vi "Config Spark Max SLOT Close Loop HW Get Set.vi"(4 "PIDF Slot (0)":i32, 6 "Get(f) Set(t)":bool, 7 "SparkMax Slot CL":T1={"Gains"={"P"=0.1, "I"=0.0, "D"=0.0, "F"=0.0}, "I Zone"=1.0, "Peak Out -1 0 1"={"High"=0.0, "Low"=0.0}, "Max I Accu"=0.0} {"Gains"."F" format="%#.8f"; "Gains"."D" format="%#.8f"; "Gains"."I" format="%#.8f"; "Gains"."P" format="%#.8f"; "Peak Out -1 0 1"."Low" format="%#.8f"; "Peak Out -1 0 1"."High" format="%#.8f"}, 8 "Error":errorcluster, 11 "Drive Refs":T4) -> (0 "Error Out":errorcluster, 3 "Drive Refs Out":T4, 5 "SparkMax Slot CL Out":T1={"Gains"={"P"=0.1, "I"=0.0, "D"=0.0, "F"=0.0}, "I Zone"=1.0, "Peak Out -1 0 1"={"High"=0.0, "Low"=0.0}, "Max I Accu"=0.0} {"Gains"."F" format="%#.8f"; "Gains"."D" format="%#.8f"; "Gains"."I" format="%#.8f"; "Gains"."P" format="%#.8f"; "Peak Out -1 0 1"."Low" format="%#.8f"; "Peak Out -1 0 1"."High" format="%#.8f"})   [LabVIEW 2020, in "Swerve AM_ACT.lvlib"]
uses:
  Swerve AM_ACT.lvlib
  <vilib>/Rock Robotics/WPI/MotorControl/WPI_MotorControlDeviceRef.ctl
  <vilib>/Rock Robotics/WPI/MotorControl/WPI_MotorControlType.ctl
  <vilib>/Rock Robotics/SystemInterfaces/DIO/FPGA_DIOPWMChannel.ctl
  <vilib>/Rock Robotics/WPI/PWM/WPI_PWMDeadband.ctl
  <vilib>/Rock Robotics/SystemInterfaces/DIO/FPGA_DIOChannel.ctl
  Shared Code/TypeDefs/Cluster_Spark MAX SLOT PID Config.ctl
  Shared Code/TypeDefs/Cluster_PID Gains.ctl
  Shared Code/TypeDefs/Cluster_High-Low.ctl
  Shared Code/TypeDefs/Cluster_SRX SLOT PID Config.ctl
  <vilib>/Utility/Data Type/NI_Data Type.lvlib
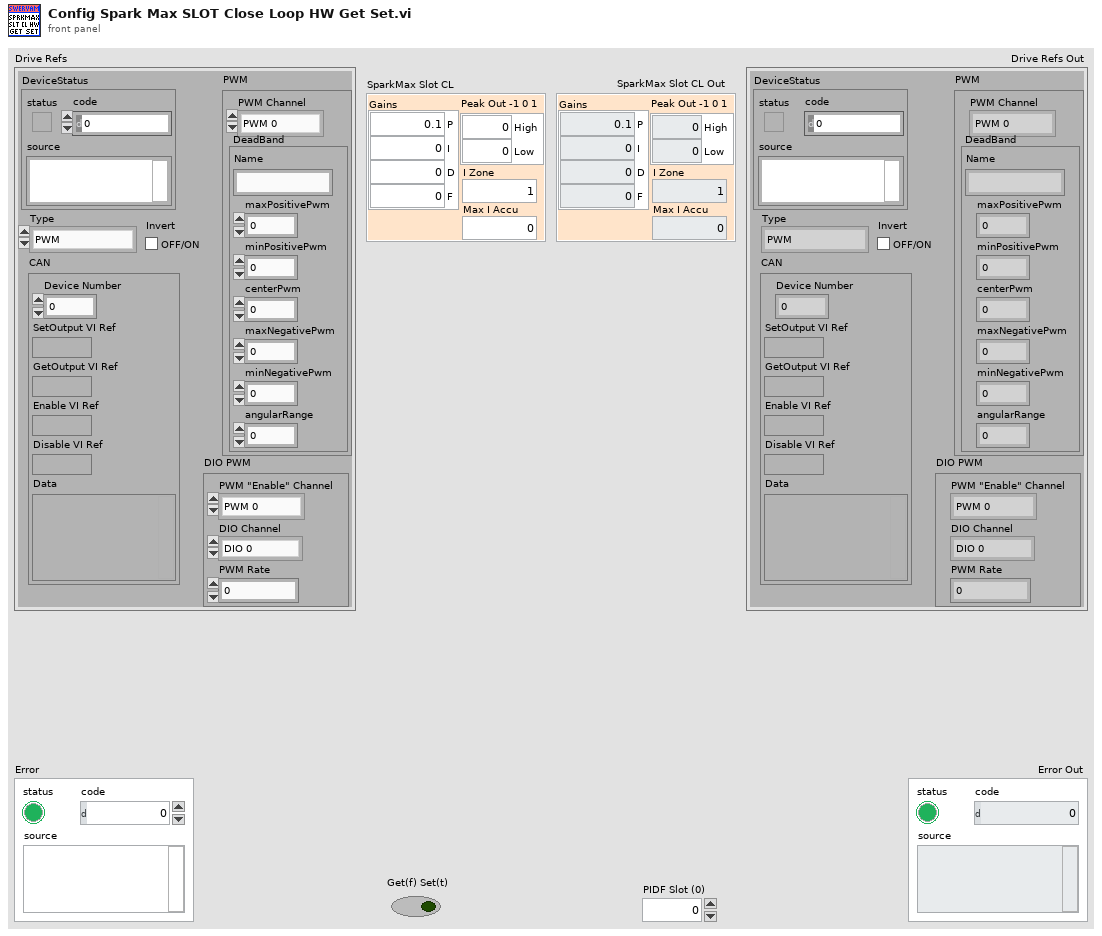
[diagram p1: front panel]
types:
  T1 = typedef "Cluster_Spark MAX SLOT PID Config.ctl" = cluster{"Gains":T2, "I Zone":dbl, "Peak Out -1 0 1":T3, "Max I Accu":dbl}
  T2 = typedef "Cluster_PID Gains.ctl" = cluster{"P":dbl, "I":dbl, "D":dbl, "F":dbl}
  T3 = typedef "Cluster_High-Low.ctl" = cluster{"High":dbl, "Low":dbl}
  T4 = typedef "WPI_MotorControlDeviceRef.ctl" = cluster{"DeviceStatus":errorcluster, "Type":T5, "PWM":cluster{"PWM Channel":T6, "DeadBand":T7}, "CAN":cluster{"Device Number":u8, "SetOutput VI Ref":variant, "GetOutput VI Ref":variant, "Enable VI Ref":variant, "Disable VI Ref":variant, "Data":variant}, "Invert":bool, "DIO PWM":cluster{"PWM \"Enable\" Channel":T6, "DIOChannel":T8, "PWM Rate":dbl}}
  T5 = typedef "WPI_MotorControlType.ctl" = enum16{"PWM", "CAN", "DIO PWM"}
  T6 = typedef "FPGA_DIOPWMChannel.ctl" = enum8{"PWM 0", "PWM 1", "PWM 2", "PWM 3", "PWM 4", "PWM 5", "PWM 6", "PWM 7", "PWM 8", "PWM 9", "PWM MXP 0", "PWM MXP 1", "PWM MXP 2", "PWM MXP 3", "PWM MXP 4", "PWM MXP 5", "PWM MXP 6", "PWM MXP 7", "PWM MXP 8", "PWM MXP 9", "Invalid"}
  T7 = typedef "WPI_PWMDeadband.ctl" = cluster{"Name":string, "maxPositivePwm":i32, "minPositivePwm":i32, "centerPwm":i32, "maxNegativePwm":i32, "minNegativePwm":i32, "angularRange":u16}
  T8 = typedef "FPGA_DIOChannel.ctl" = enum8{"DIO 0", "DIO 1", "DIO 2", "DIO 3", "DIO 4", "DIO 5", "DIO 6", "DIO 7", "DIO 8", "DIO 9", "DIO MXP 0", "DIO MXP 1", "DIO MXP 2", "DIO MXP 3", "DIO MXP 4", "DIO MXP 5", "DIO MXP 6", "DIO MXP 7", "DIO MXP 8", "DIO MXP 9", "DIO MXP 10", "DIO MXP 11", "DIO MXP 12", "DIO MXP 13", "DIO MXP 14", "DIO MXP 15", "SPI Port CS1", "SPI Port CS2", "SPI Port CS3", "SPI Port MISO", "SPI Port MOSI", "Invalid"}
  T9 = typedef "Cluster_SRX SLOT PID Config.ctl" = cluster{"Gains":T2, "Error Allowed":dbl, "I Zone":dbl, "Peak Out 0-1":dbl, "Max I Accu":dbl}
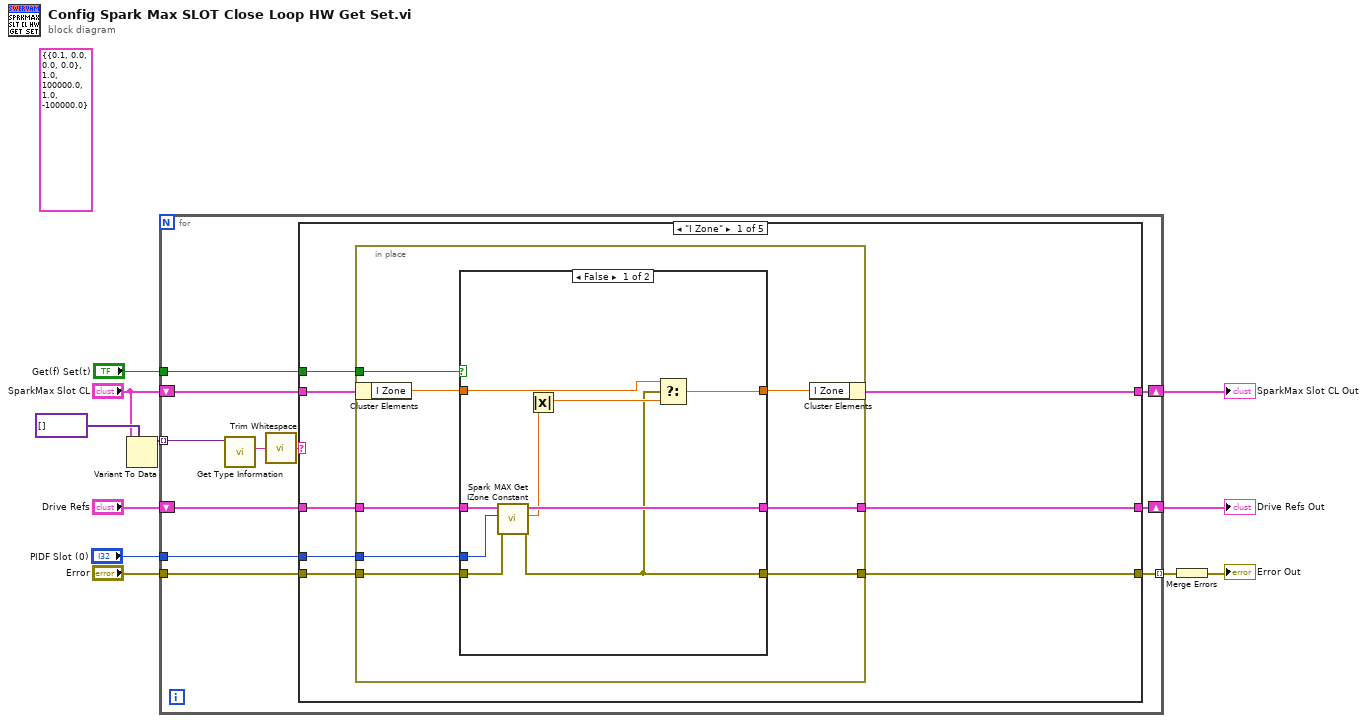
[diagram p0: block diagram]
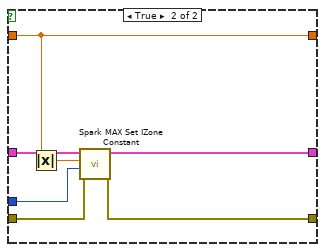
[diagram p2: hidden frame]
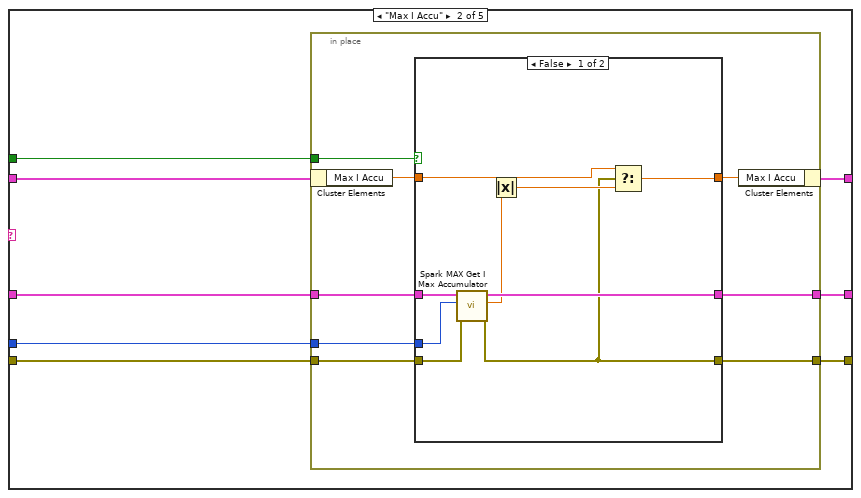
[diagram p3: hidden frame]
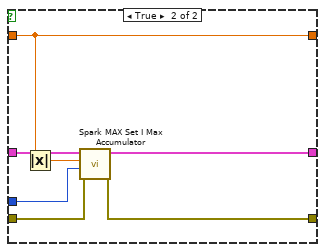
[diagram p4: hidden frame]
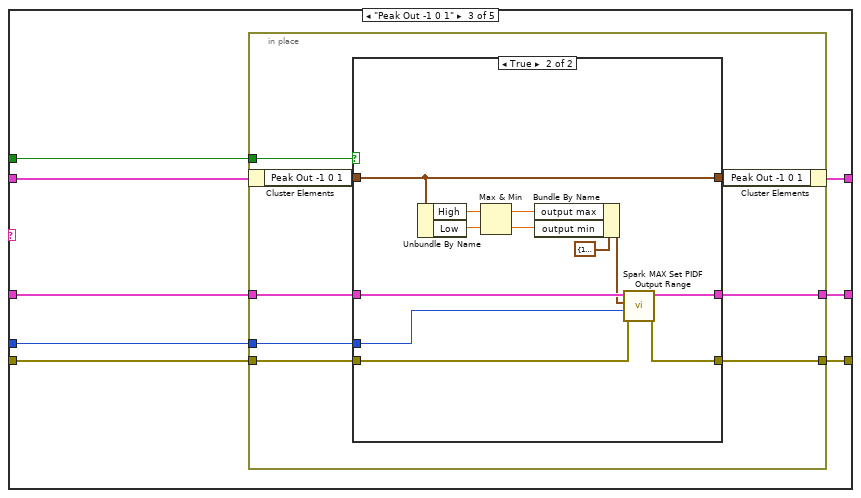
[diagram p5: hidden frame]
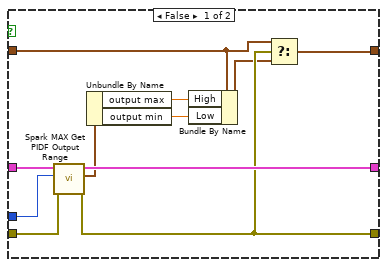
[diagram p6: hidden frame]
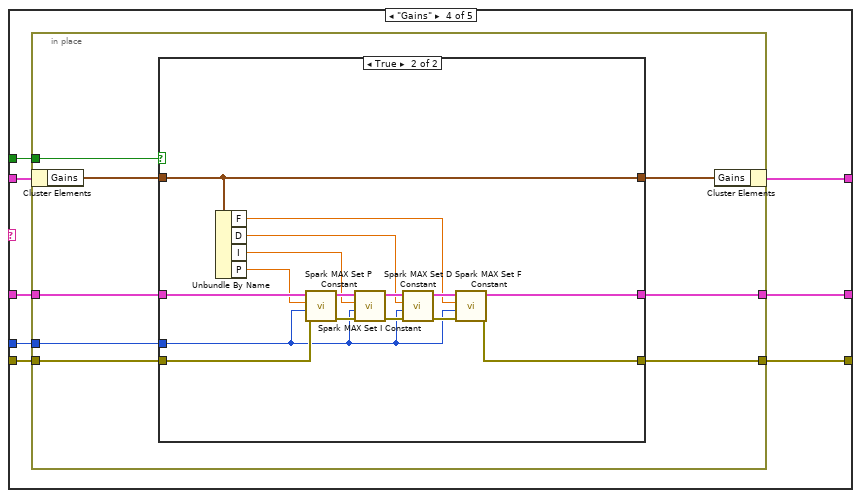
[diagram p7: hidden frame]
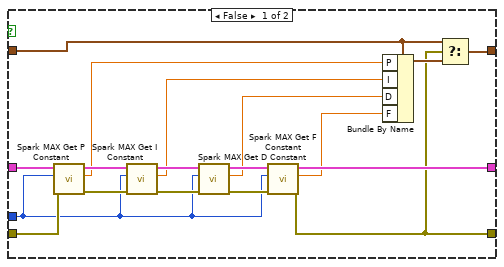
[diagram p8: hidden frame]
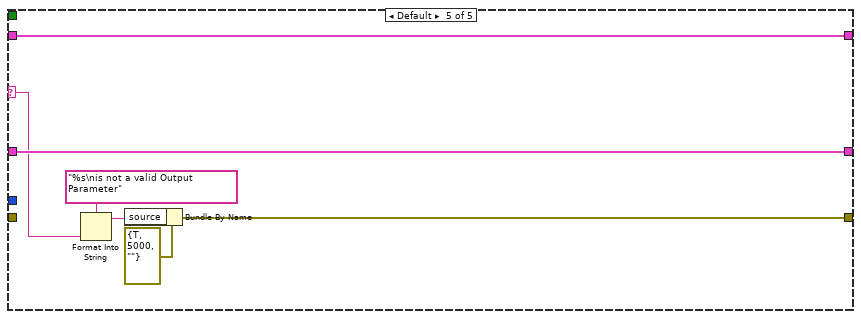
[diagram p9: hidden frame]
diagram:
  (unwired) T9 {"Gains"={"P"=0.1, "I"=0.0, "D"=0.0, "F"=0.0}, "Error Allowed"=1.0, "I Zone"=100000.0, "Peak Out 0-1"=1.0, "Max I Accu"=-100000.0} ("SparkMax Output")
  n1 = Variant To Data(type=variant[] [], Variant="SparkMax Slot CL") -> (data=w6:variant[])  [unwired: 1 in, 1 out]
  n2 = for {
    shift-right: [w13] -> w11
    shift-left: "SparkMax Slot CL" -> [w19]
    shift-right: [w14] -> w9
    shift-left: "Drive Refs" -> [w18]
    tunnel: "Get(f) Set(t)" -> [w17]
    tunnel: w6 -> [w21] mode=indexing
    tunnel: "Error" -> [w16]
    tunnel: [w15] -> w3 mode=indexing
    tunnel: "PIDF Slot (0)" -> [w12]
    n3 = call <vilib>:"Get Type Information.vi"("variant"=w21) -> ("name"=w22:string)  [unwired: 6 in, 4 out]
    n4 = call <vilib>:"Trim Whitespace.vi"("string"=w22) -> ("trimmed string"=w20:string)  [unwired: 1 in]
    n5 = case shown="\"I Zone\"" w20 {
      selector: w20 -> [_ _ _ _ w180]
      tunnel: w19 -> [w30 w62 w94 w133 w182]
      tunnel: w18 -> [w26 w58 w90 w129 w181]
      tunnel: w17 -> [w29 w61 w93 w132 _]
      tunnel: w16 -> [w28 w60 w92 w131 _]
      tunnel: [w27 w59 w91 w130 w178] -> w15
      tunnel: [w25 w57 w89 w128 w181] -> w14
      tunnel: [w24 w56 w88 w127 w182] -> w13
      tunnel: w12 -> [w23 w55 w87 w126 _]
      frame "I Zone" {
        n6 = in-place {
          in-place-border: w29 -> [w38]
          in-place-border: w28 -> [w36]
          in-place-border: [w35] -> w27
          in-place-border: w26 -> [w34]
          in-place-border: [w33] -> w25
          in-place-border: w23 -> [w31]
          n7 = in-place-cluster #1(w30) -> ("I Zone"=w37:dbl)
          n8 = case shown="False" w38 {
            tunnel: w37 -> [w46 w54]
            tunnel: w36 -> [w40 w49]
            tunnel: [w39 w48] -> w35
            tunnel: w34 -> [w43 w53]
            tunnel: [w42 w52] -> w33
            tunnel: [w47 w54] -> w32
            tunnel: w31 -> [w44 w50]
            frame False {
              n9 = call <vilib>:"Spark MAX Get IZone Constant.vi"("error in (no error)"=w40, "PIDF Slot (0)"=w44, "MotorControlDeviceRef in"=w43) -> ("error out"=w39:errorcluster, "IZone"=w41:dbl, "MotorControlDeviceRef out"=w42:T4)  [unwired: 6 in]
              n10 = Absolute Value(x=w41) -> (abs(x)=w45:dbl)
              n11 = Select(t=w46, s=w39, f=w45) -> (s? t:f=w47:dbl)
            }
            frame True {
              n12 = Absolute Value(x=w54) -> (abs(x)=w51:dbl)
              n13 = call <vilib>:"Spark MAX Set IZone Constant.vi"("error in"=w49, "PIDF Slot"=w50, "IZone"=w51, "MotorControlDeviceRef"=w53) -> ("error out"=w48:errorcluster, "MotorControlDeviceRef"=w52:T4)  [unwired: 6 in]
            }
          }
          n14 = in-place-cluster #1("I Zone"=w32) -> (w24:T1)
        }
      }
      frame "Max I Accu" {
        n15 = in-place {
          in-place-border: w61 -> [w70]
          in-place-border: w60 -> [w68]
          in-place-border: [w67] -> w59
          in-place-border: w58 -> [w66]
          in-place-border: [w65] -> w57
          in-place-border: w55 -> [w63]
          n16 = in-place-cluster #2(w62) -> ("Max I Accu"=w69:dbl)
          n17 = case shown="False" w70 {
            tunnel: w69 -> [w78 w86]
            tunnel: w68 -> [w71 w81]
            tunnel: [w73 w80] -> w67
            tunnel: w66 -> [w76 w85]
            tunnel: [w75 w84] -> w65
            tunnel: [w79 w86] -> w64
            tunnel: w63 -> [w72 w82]
            frame False {
              n18 = call <vilib>:"Spark MAX Get I Max Accumulator.vi"("error in (no error)"=w71, "PIDF Slot (0)"=w72, "MotorControlDeviceRef in"=w76) -> ("error out"=w73:errorcluster, "Max Accumulator"=w74:dbl, "MotorControlDeviceRef out"=w75:T4)  [unwired: 6 in]
              n19 = Absolute Value(x=w74) -> (abs(x)=w77:dbl)
              n20 = Select(t=w78, s=w73, f=w77) -> (s? t:f=w79:dbl)
            }
            frame True {
              n21 = Absolute Value(x=w86) -> (abs(x)=w83:dbl)
              n22 = call <vilib>:"Spark MAX Set I Max Accumulator.vi"("error in"=w81, "PIDF Slot (0)"=w82, "Max I Accumulator"=w83, "MotorControlDeviceRef"=w85) -> ("error out"=w80:errorcluster, "MotorControlDeviceRef"=w84:T4)  [unwired: 6 in]
            }
          }
          n23 = in-place-cluster #2("Max I Accu"=w64) -> (w56:T1)
        }
      }
      frame "Peak Out -1 0 1" {
        n24 = in-place {
          in-place-border: w93 -> [w102]
          in-place-border: w92 -> [w100]
          in-place-border: [w99] -> w91
          in-place-border: w90 -> [w98]
          in-place-border: [w97] -> w89
          in-place-border: w87 -> [w95]
          n25 = in-place-cluster #3(w94) -> ("Peak Out -1 0 1"=w101:T3)
          n26 = case shown="True" w102 {
            tunnel: w101 -> [w106 w118]
            tunnel: w100 -> [w110 w123]
            tunnel: [w107 w122] -> w99
            tunnel: w98 -> [w112 w125]
            tunnel: [w111 w124] -> w97
            tunnel: [w113 w118] -> w96
            tunnel: w95 -> [w109 w121]
            frame False {
              n27 = call <vilib>:"Spark MAX Get PIDF Output Range.vi"("error in (no error)"=w110, "PIDF Slot (0)"=w109, "MotorControlDeviceRef in"=w112) -> ("error out"=w107:errorcluster, "output range"=w108:cluster{"output max":dbl, "output min":dbl}, "MotorControlDeviceRef out"=w111:T4)  [unwired: 6 in]
              n28 = Unbundle By Name(w108) -> ("output max"=w104:dbl, "output min"=w103:dbl)
              n29 = Bundle By Name(cluster=w106, "High"=w104, "Low"=w103) -> (w105:T3)
              n30 = Select(t=w106, s=w107, f=w105) -> (s? t:f=w113:T3)
            }
            frame True {
              n31 = Unbundle By Name(w118) -> ("High"=w117:dbl, "Low"=w115:dbl)
              n32 = Max & Min(x=w117, y=w115) -> (max(x,y)=w116:dbl, min(x,y)=w114:dbl)
              n33 = Bundle By Name(cluster=cluster{"output max":dbl, "output min":dbl} {"output max"=1.0, "output min"=-1.0} ("output range"), "output max"=w116, "output min"=w114) -> (w119:cluster{"output max":dbl, "output min":dbl})
              n34 = call <vilib>:"Spark MAX Set PIDF Output Range.vi"("error in"=w123, "PIDF Slot (0)"=w121, "output range"=w119, "MotorControlDeviceRef"=w125) -> ("error out"=w122:errorcluster, "MotorControlDeviceRef"=w124:T4)  [unwired: 6 in]
            }
          }
          n35 = in-place-cluster #3("Peak Out -1 0 1"=w96) -> (w88:T1)
        }
      }
      frame "Gains" {
        n36 = in-place {
          in-place-border: w132 -> [w141]
          in-place-border: w131 -> [w139]
          in-place-border: [w138] -> w130
          in-place-border: w129 -> [w137]
          in-place-border: [w136] -> w128
          in-place-border: w126 -> [w134]
          n37 = in-place-cluster #4(w133) -> ("Gains"=w140:T2)
          n38 = case shown="True" w141 {
            tunnel: w140 -> [w158 w165]
            tunnel: w139 -> [w147 w166]
            tunnel: [w148 w167] -> w138
            tunnel: w137 -> [w153 w172]
            tunnel: [w152 w168] -> w136
            tunnel: [w159 w165] -> w135
            tunnel: w134 -> [w142 w164]
            frame False {
              n39 = call <vilib>:"Spark MAX Get P Constant.vi"("error in (no error)"=w147, "PIDF Slot (0)"=w142, "MotorControlDeviceRef in"=w153) -> ("error out"=w151:errorcluster, "kP"=w146:dbl, "MotorControlDeviceRef out"=w156:T4)  [unwired: 6 in]
              n40 = call <vilib>:"Spark MAX Get I Constant.vi"("error in (no error)"=w151, "PIDF Slot (0)"=w142, "MotorControlDeviceRef in"=w156) -> ("error out"=w150:errorcluster, "kI"=w145:dbl, "MotorControlDeviceRef out"=w155:T4)  [unwired: 6 in]
              n41 = call <vilib>:"Spark MAX Get D Constant.vi"("error in (no error)"=w150, "PIDF Slot (0)"=w142, "MotorControlDeviceRef in"=w155) -> ("error out"=w149:errorcluster, "kD"=w144:dbl, "MotorControlDeviceRef out"=w154:T4)  [unwired: 6 in]
              n42 = call <vilib>:"Spark MAX Get F Constant.vi"("error in (no error)"=w149, "PIDF Slot (0)"=w142, "MotorControlDeviceRef in"=w154) -> ("error out"=w148:errorcluster, "kF"=w143:dbl, "MotorControlDeviceRef out"=w152:T4)  [unwired: 6 in]
              n43 = Bundle By Name(cluster=w158, "P"=w146, "I"=w145, "D"=w144, "F"=w143) -> (w157:T2)
              n44 = Select(t=w158, s=w148, f=w157) -> (s? t:f=w159:T2)
            }
            frame True {
              n45 = Unbundle By Name(w165) -> ("F"=w160:dbl, "D"=w161:dbl, "I"=w162:dbl, "P"=w163:dbl)
              n46 = call <vilib>:"Spark MAX Set P Constant.vi"("error in"=w166, "PIDF Slot"=w164, "kP"=w163, "MotorControlDeviceRef"=w172) -> ("error out"=w175:errorcluster, "MotorControlDeviceRef"=w171:T4)  [unwired: 6 in]
              n47 = call <vilib>:"Spark MAX Set I Constant.vi"("error in"=w175, "PIDF Slot"=w164, "kI"=w162, "MotorControlDeviceRef"=w171) -> ("error out"=w174:errorcluster, "MotorControlDeviceRef"=w170:T4)  [unwired: 6 in]
              n48 = call <vilib>:"Spark MAX Set D Constant.vi"("error in"=w174, "PIDF Slot"=w164, "kD"=w161, "MotorControlDeviceRef"=w170) -> ("error out"=w173:errorcluster, "MotorControlDeviceRef"=w169:T4)  [unwired: 6 in]
              n49 = call <vilib>:"Spark MAX Set F Constant.vi"("error in"=w173, "PIDF Slot"=w164, "kF"=w160, "MotorControlDeviceRef"=w169) -> ("error out"=w167:errorcluster, "MotorControlDeviceRef"=w168:T4)  [unwired: 6 in]
            }
          }
          n50 = in-place-cluster #4("Gains"=w135) -> (w127:T1)
        }
      }
      frame Default {
        n51 = Format Into String(format string="%s\nis not a valid Output Parameter", w180) -> (resulting string=w176:string)  [unwired: 2 in, 1 out]
        n52 = Bundle By Name(cluster=errorcluster {"status"=TRUE, "code"=5000, "source"=""} ("error out"), "source"=w176) -> (w178:errorcluster)
      }
    }
  }
  "Drive Refs Out" <- w9
  "SparkMax Slot CL Out" <- w11
  n53 = Merge Errors(w3) -> (→"Error Out":errorcluster)
